vi "5492_WPI_RobotDriveOpen4MotorWithTalonSRX_Position.vi"(0 "Front Left Motor":T1=enum."Invalid", 1 "Front Left Motor Inverted":bool, 3 "Front Right Motor Inverted":bool, 5 "Front Right Motor":T1=enum."Invalid", 7 "Back Left Motor":T1=enum."Invalid", 9 "Back Right Motor":T1=enum."Invalid", 11 "error in (no error)":errorcluster, 12 "Back Left Motor Inverted":bool, 14 "Back Right Motor Inverted":bool) -> (4 "RobotDriveDevRef":T2={"DevStatus"={"status"=FALSE, "code"=0, "source"=""}, "Motors[]"=[], "Square Inputs"=FALSE, "Max Output"=1.0}, 15 "error out":errorcluster)   [LabVIEW 2016]
doc: "Opens a reference to the robot drive for a two-motor robot using TalonSRX motor controllers.\n\nThis software is licensed. Open the labview\\readme\\WPI Robotics Library Open Source License.txt file for more information."
uses:
  <vilib>/Rock Robotics/SystemInterfaces/DIO/FPGA_DIOPWMChannel.ctl
  <vilib>/Rock Robotics/WPI/RobotDrive/WPI_RobotDriveDevRef.ctl
  <vilib>/Rock Robotics/WPI/MotorControl/WPI_MotorControlDeviceRef.ctl
  <vilib>/Rock Robotics/WPI/MotorControl/WPI_MotorControlType.ctl
  <vilib>/Rock Robotics/WPI/PWM/WPI_PWMDeadband.ctl
  <vilib>/Rock Robotics/WPI/SafetyOutput/WPI_SafetyOutputConfigMenu.ctl
  <vilib>/Rock Robotics/WPI/ThirdParty/CanMotor/TalonSRX/WPI_CANTalonSRX_APIControlMode.ctl
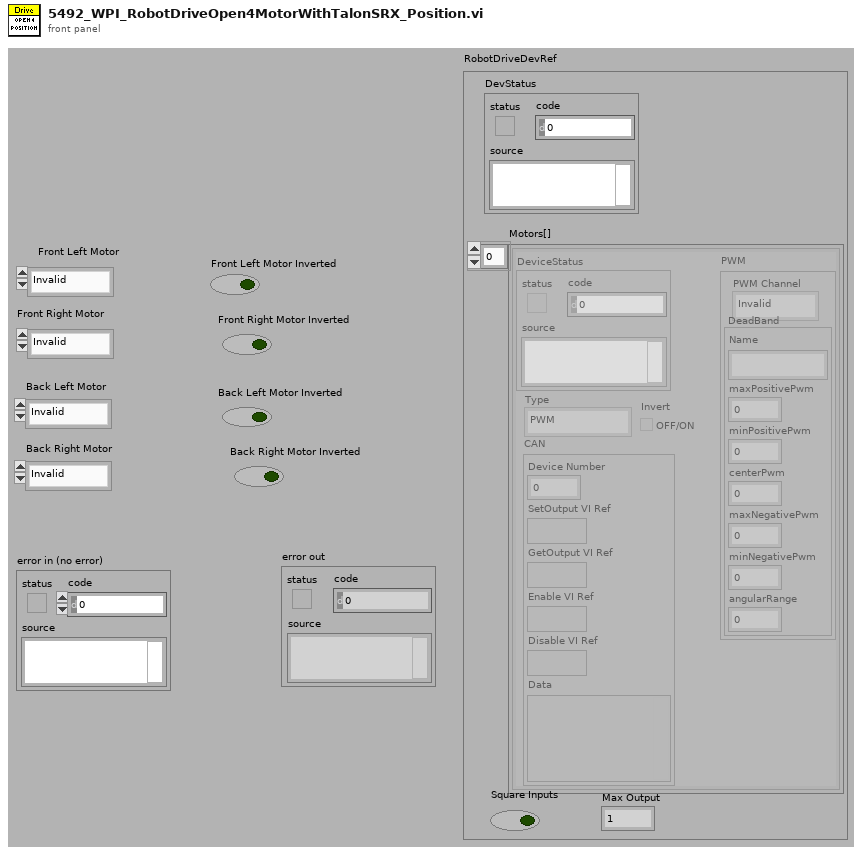
[diagram p1: front panel]
types:
  T1 = typedef "FPGA_DIOPWMChannel.ctl" = enum8{"PWM 0", "PWM 1", "PWM 2", "PWM 3", "PWM 4", "PWM 5", "PWM 6", "PWM 7", "PWM 8", "PWM 9", "PWM MXP 0", "PWM MXP 1", "PWM MXP 2", "PWM MXP 3", "PWM MXP 4", "PWM MXP 5", "PWM MXP 6", "PWM MXP 7", "PWM MXP 8", "PWM MXP 9", "Invalid"}
  T2 = typedef "WPI_RobotDriveDevRef.ctl" = cluster{"DevStatus":errorcluster, "Motors[]":T3[], "Square Inputs":bool, "Max Output":dbl}
  T3 = typedef "WPI_MotorControlDeviceRef.ctl" = cluster{"DeviceStatus":errorcluster, "Type":T4, "PWM":cluster{"PWM Channel":T1, "DeadBand":T5}, "CAN":cluster{"Device Number":u8, "SetOutput VI Ref":variant, "GetOutput VI Ref":variant, "Enable VI Ref":variant, "Disable VI Ref":variant, "Data":variant}, "Invert":bool}
  T4 = typedef "WPI_MotorControlType.ctl" = enum16{"PWM", "CAN"}
  T5 = typedef "WPI_PWMDeadband.ctl" = cluster{"Name":string, "maxPositivePwm":i32, "minPositivePwm":i32, "centerPwm":i32, "maxNegativePwm":i32, "minNegativePwm":i32, "angularRange":u16}
  T6 = typedef "WPI_CANTalonSRX_APIControlMode.ctl" = enum8{"Percent VBus", "Speed", "Position", "Slave", "Unchanged / Invalid", "Voltage Compensation", "Current", "Motion Profile", "Motion Magic"}
  T7 = typedef "WPI_SafetyOutputConfigMenu.ctl" = enum16{"Enable", "Disable"}
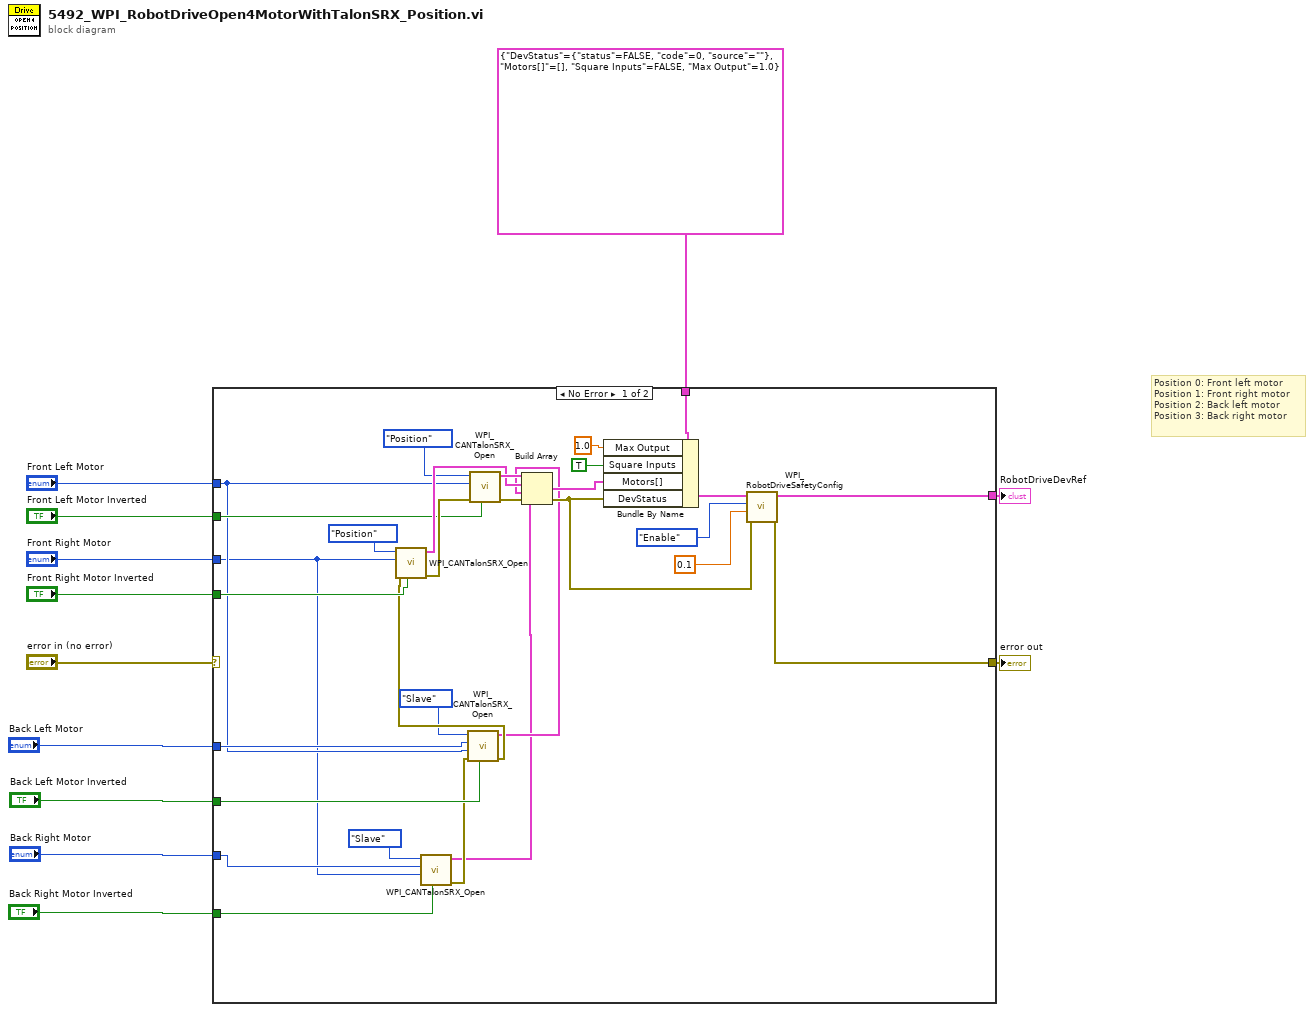
[diagram p0: block diagram]
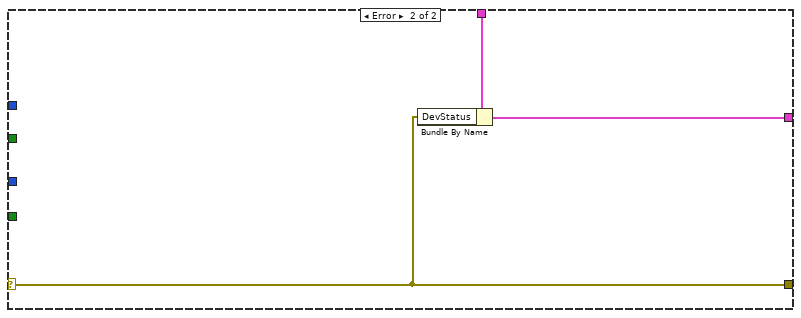
[diagram p2: hidden frame]
diagram:
  # "Position 0: Front left motor\nPosition 1: Front right motor\nPosition 2: Back left motor\nPosition 3: Back right motor"
  n1 = case shown="No Error" "error in (no error)" {
    selector: "error in (no error)" -> [_ w42]
    tunnel: "Front Left Motor" -> [w14 _]
    tunnel: "Front Right Motor" -> [w13 _]
    tunnel: [w29 w44] -> w5
    tunnel: "Front Left Motor Inverted" -> [w35 _]
    tunnel: "Front Right Motor Inverted" -> [w36 _]
    tunnel: T2 {"DevStatus"={"status"=FALSE, "code"=0, "source"=""}, "Motors[]"=[], "Square Inputs"=FALSE, "Max Output"=1.0} ("RobotDriveDevRef") -> [w40 w43]
    tunnel: [w30 w42] -> w7
    tunnel: "Back Left Motor" -> [w17 _]
    tunnel: "Back Right Motor" -> [w16 _]
    tunnel: "Back Left Motor Inverted" -> [w26 _]
    tunnel: "Back Right Motor Inverted" -> [w25 _]
    frame No Error {
      n2 = call <vilib>:"WPI_CANTalonSRX_Open.vi"("Invert"=w25, "Master Device Number"=w13, "Device Number"=w16, "Control Mode"=WPI_CANTalonSRX_APIControlMode."Slave") -> ("error out"=w24:errorcluster, "CAN Talon SRX Ref"=w21:T3)  [unwired: 6 in]
      n3 = call <vilib>:"WPI_CANTalonSRX_Open.vi"("Invert"=w26, "error in"=w24, "Master Device Number"=w14, "Device Number"=w17, "Control Mode"=WPI_CANTalonSRX_APIControlMode."Slave") -> ("error out"=w23:errorcluster, "CAN Talon SRX Ref"=w22:T3)  [unwired: 5 in]
      n4 = call <vilib>:"WPI_CANTalonSRX_Open.vi"("Invert"=w36, "error in"=w23, "Device Number"=w13, "Control Mode"=WPI_CANTalonSRX_APIControlMode."Position") -> ("error out"=w39:errorcluster, "CAN Talon SRX Ref"=w37:T3)  [unwired: 6 in]
      n5 = call <vilib>:"WPI_CANTalonSRX_Open.vi"("Invert"=w35, "error in"=w39, "Device Number"=w14, "Control Mode"=WPI_CANTalonSRX_APIControlMode."Position") -> ("error out"=w31:errorcluster, "CAN Talon SRX Ref"=w38:T3)  [unwired: 6 in]
      n6 = Build Array(w38, w37, w22, w21) -> (w41:T3[])
      n7 = Bundle By Name(cluster=w40, "Max Output"=1.0, "Square Inputs"=TRUE, "Motors[]"=w41, "DevStatus"=w31) -> (w33:T2)
      n8 = call <vilib>:"WPI_RobotDriveSafetyConfig.vi"("error in (no error)"=w31, "timeout (s)"=0.1, "mode"=WPI_SafetyOutputConfigMenu."Enable", "RobotDriveDevRef"=w33) -> ("error out"=w30:errorcluster, "RobotDriveDevRef"=w29:T2)  [unwired: 6 out]
    }
    frame Error {
      n9 = Bundle By Name(cluster=w43, "DevStatus"=w42) -> (w44:T2)
    }
  }
  "RobotDriveDevRef" <- w5
  "error out" <- w7
